vi "ERD Send Receive Example.vi"() -> ()   [LabVIEW 2016]
uses:
  Save File/File Setup (Public)/Type Definition/Save File DOE LabView Program.ctl
  type defs/ERD Read Data Out.ctl
  type defs/ERD Read Data In.ctl
  type defs/Data Type.ctl
  type defs/Source_Destination.ctl
  <vilib>/Utility/file.llb/Write To Spreadsheet File (string).vi
  library/GEA2_Toolkit.lvlib
  Save File/File Setup.lvlib
panel:
  out "Output Data Send":T1[](array[typedef]) {"ERD Number" format="%.0x"}
  in  "ERD to Send":T2[](array[typedef]) {"ERD Number" format="%.0x"}
  in  "Read ERD 2":bool
  in  "Add Date and Time":bool=TRUE
  out "Rate":dbl
  in  "#ERDs per message":i32=15
  out "ERD Data Out":T1[](array[typedef]) {"ERD Number" format="%.0x"}
  in  "ERD to Read":T2[](array[typedef]) {"ERD Number" format="%.0x"}
  out "Output Data Read":T1[](array[typedef]) {"ERD Number" format="%.0x"}
  in  "Read ERD":bool
  in  "Start Test":bool
  in  "Path":path
  in  "LV Program":T4=enum."HEWH"
  in  "Disable Classic GEA2":bool
  in  "Disable Electronic Mixing Valve (EMV) List":bool
  in  "Disable ERD":bool
  in  "Board Index":i32
  out "HEWH Appliance Data":string[][](array[string])
  in  "stop":bool
  # "HEWH Wifi Module\n0x600F - 01 Off\n0x600F - 00 On"
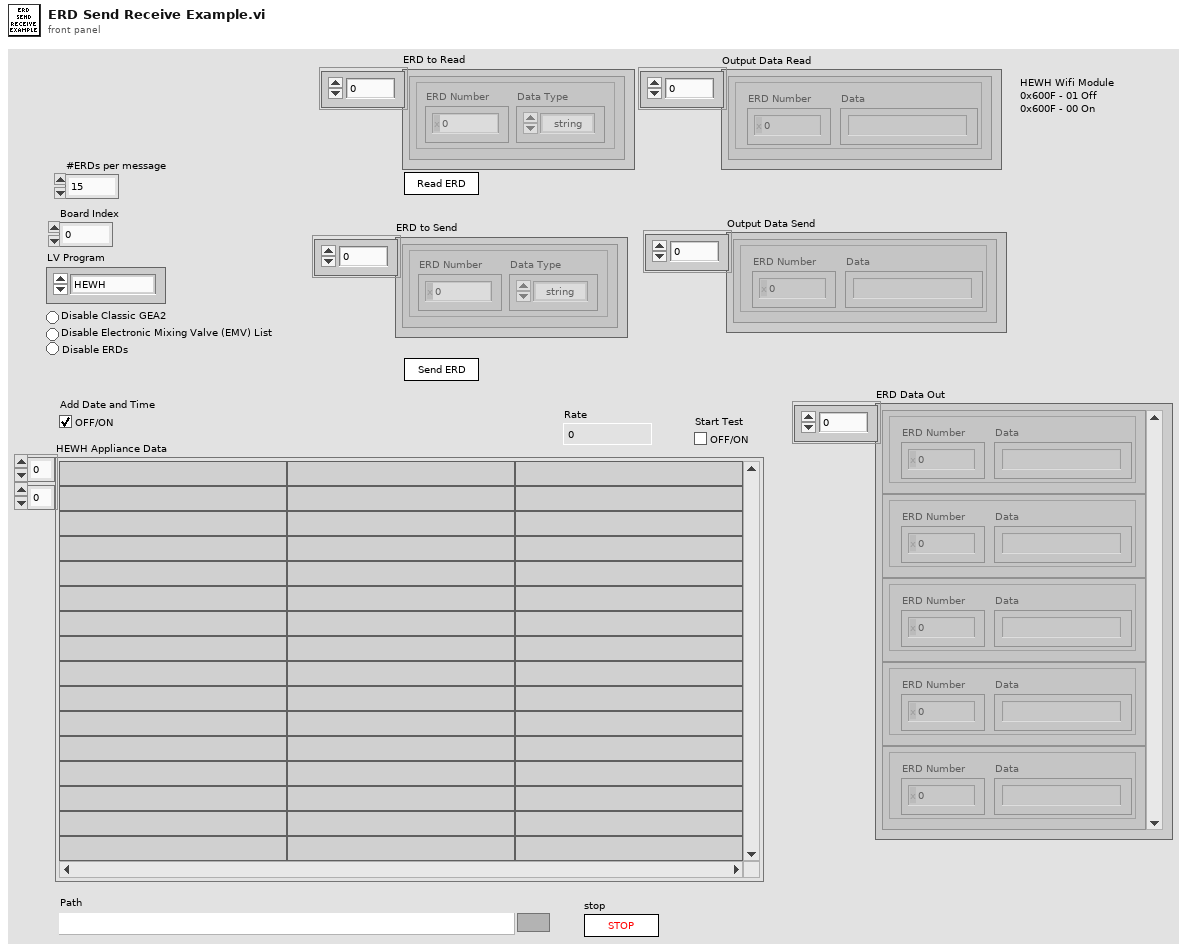
[diagram p1: front panel]
types:
  T1 = typedef "GEA2_Toolkit.lvlib/ERD Read Data Out.ctl" = cluster{"ERD Number":u16, "Data":string}
  T2 = typedef "GEA2_Toolkit.lvlib/ERD Read Data In.ctl" = cluster{"ERD Number":u16, "Data Type":T3}
  T3 = typedef "GEA2_Toolkit.lvlib/Data Type.ctl" = enum16{"string", "boolean", "uint8_t", "uint16_t", "uint32_t", "uint64_t"}
  T4 = typedef "File Setup.lvlib/Save File DOE LabView Program.ctl" = enum16{"No Name Found", "DOE Stand", "Dishwasher Kitchen", "Portable Stand", "HEWH", "Dryer", "Dryer WILT", "HCC", "PRAT", "HEWH RLT"}
  T5 = typedef "GEA2_Toolkit.lvlib/Source_Destination.ctl" = cluster{"Source":u8, "Destination":u8}
  T6 = enum32{"invalid app kind", "Development System", "Run Time System", "Student Edition", "Embedded LabVIEW", "Evaluation", "Custom"}
  T7 = enum32{"Invalid", "Standard", "Closed", "Hidden", "Minimized", "Maximized"}
  T8 = cluster{"Core":cluster{"Current VI Reference":refnum<vi>, "Close Panel on Exit?":bool}, "HEWH Appliance Data":string[][]}
  T9 = cluster{"Current VI Reference":refnum<vi>, "Close Panel on Exit?":bool}
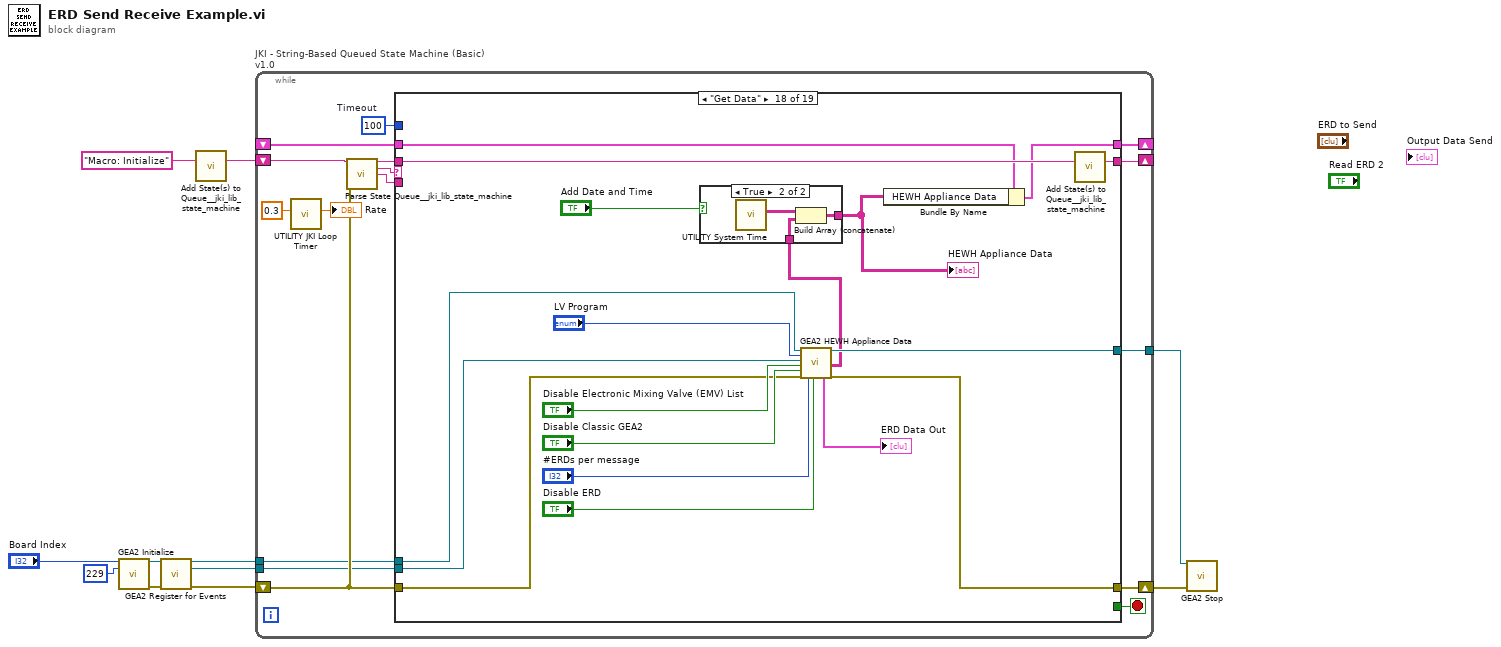
[diagram p0: block diagram]
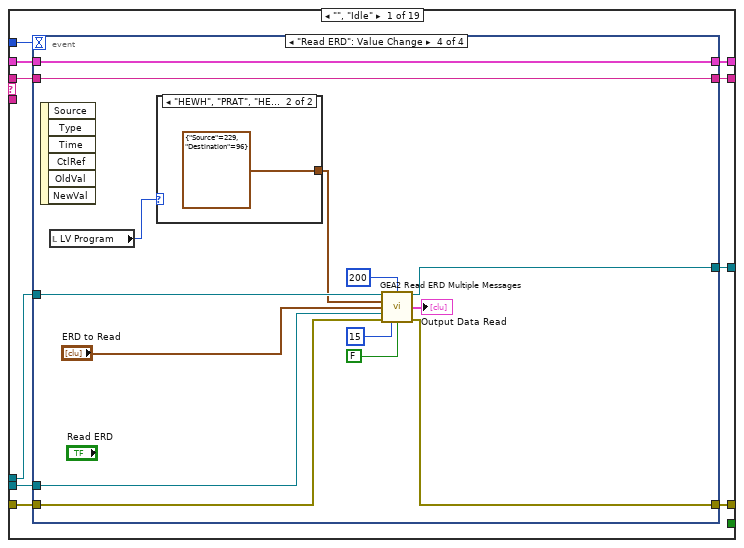
[diagram p2: hidden frame]
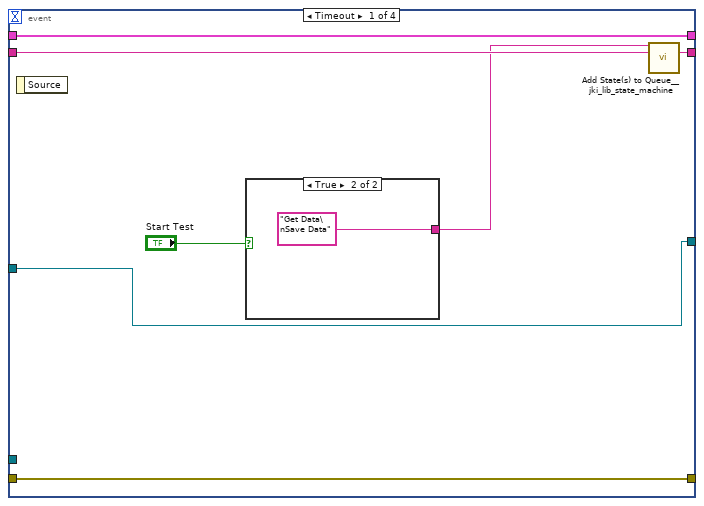
[diagram p3: hidden frame]
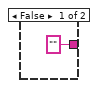
[diagram p4: hidden frame]
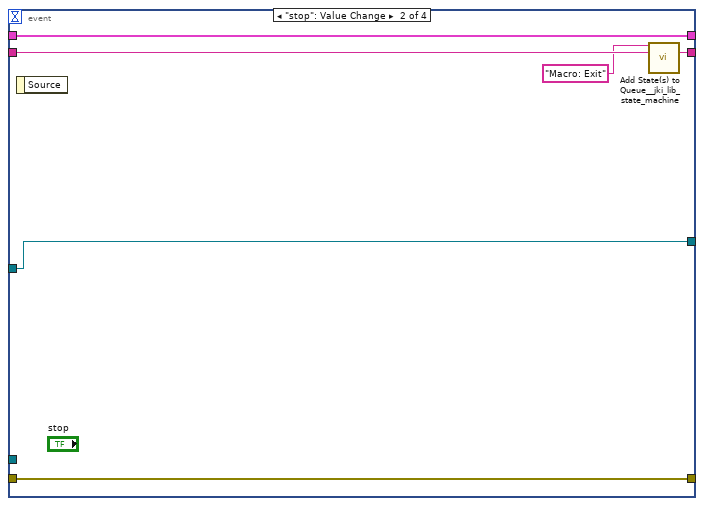
[diagram p5: hidden frame]
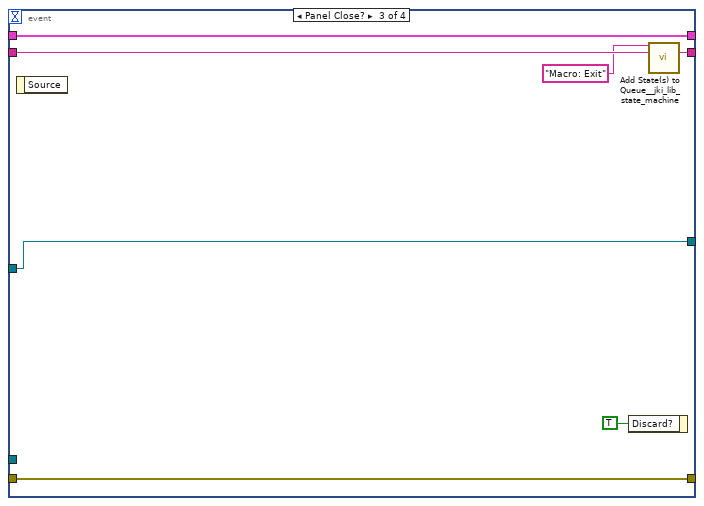
[diagram p6: hidden frame]
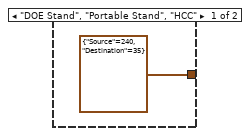
[diagram p7: hidden frame]
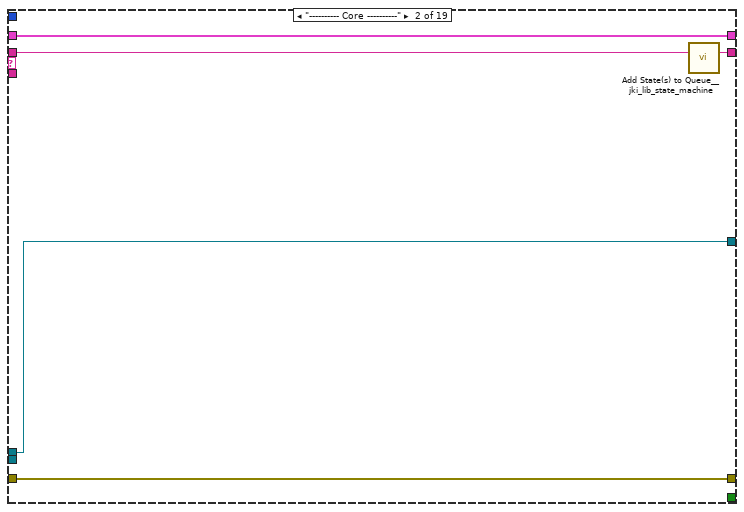
[diagram p8: hidden frame]
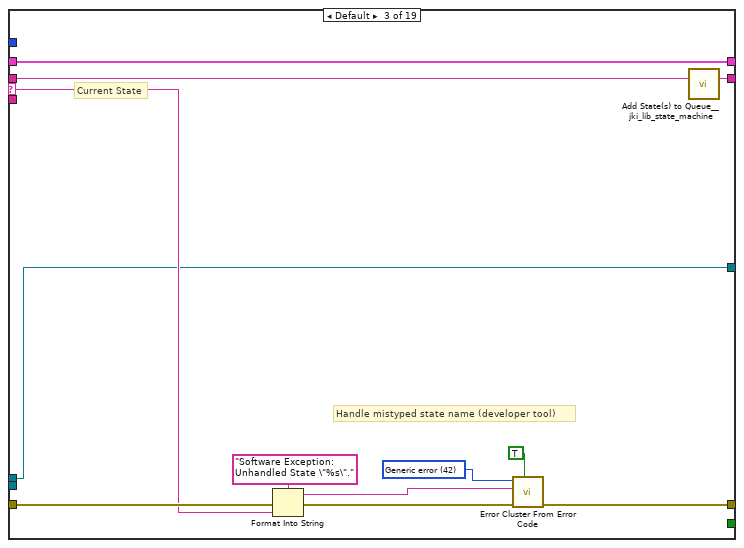
[diagram p9: hidden frame]
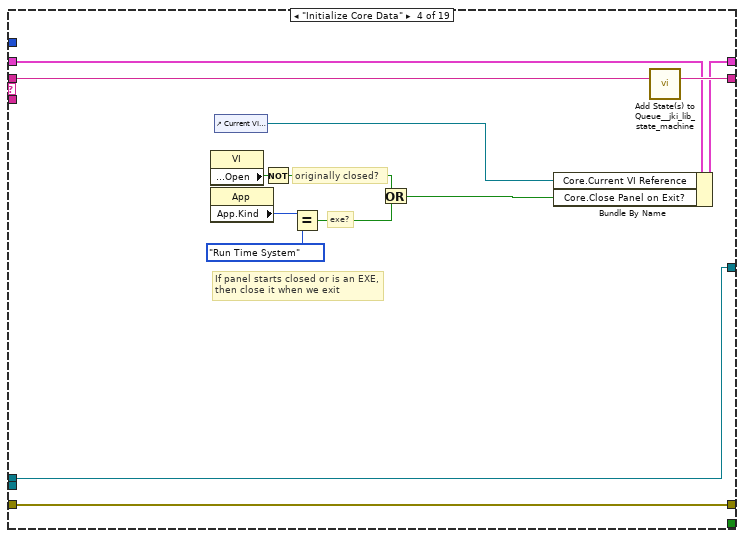
[diagram p10: hidden frame]
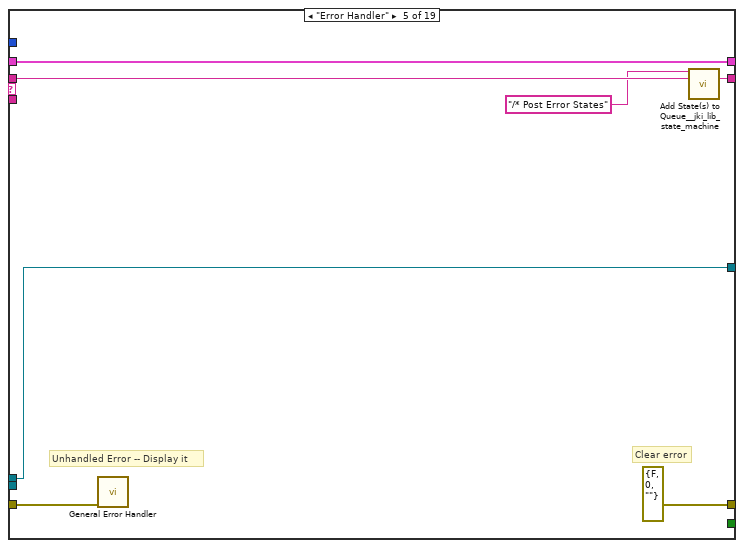
[diagram p11: hidden frame]
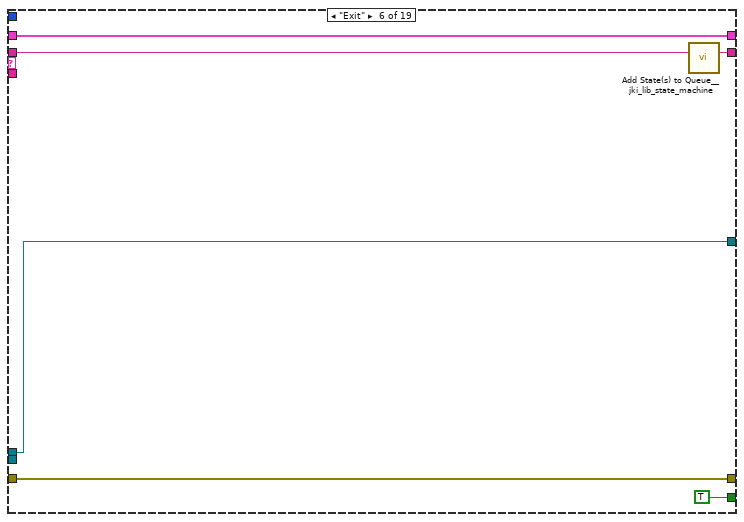
[diagram p12: hidden frame]
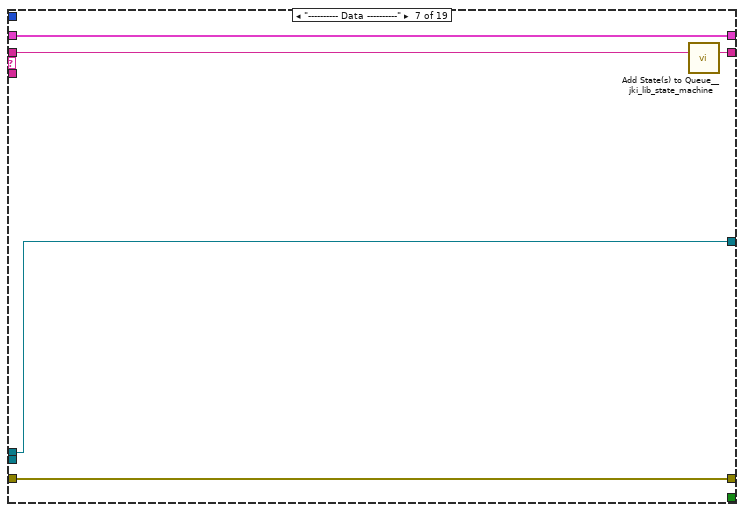
[diagram p13: hidden frame]
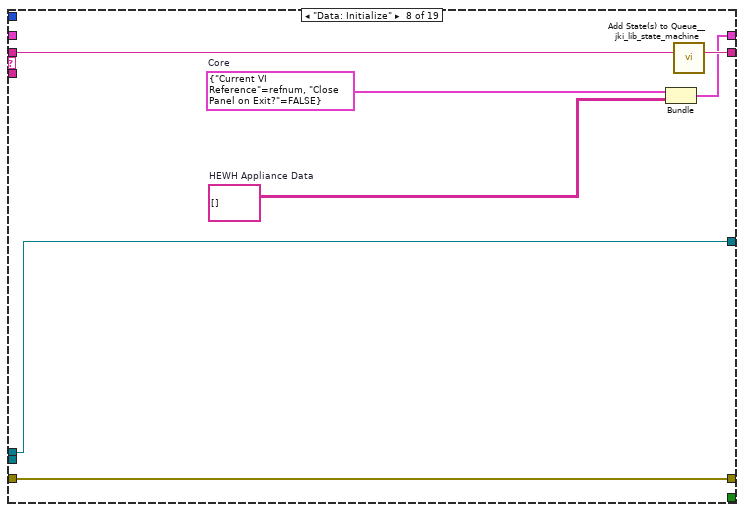
[diagram p14: hidden frame]
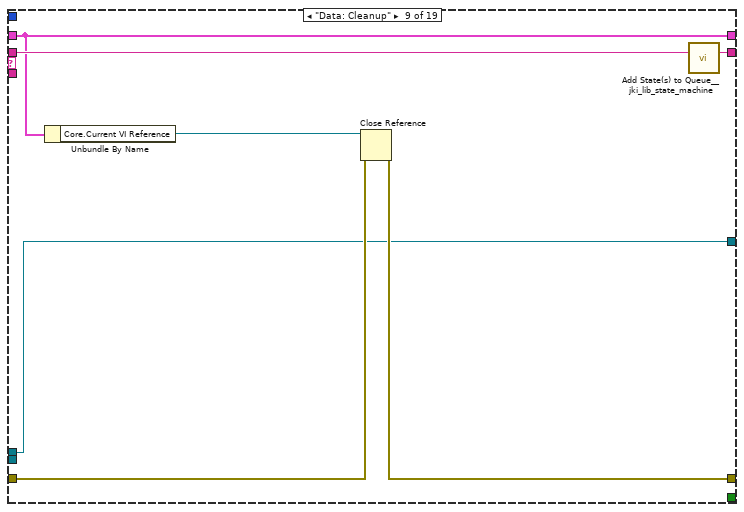
[diagram p15: hidden frame]
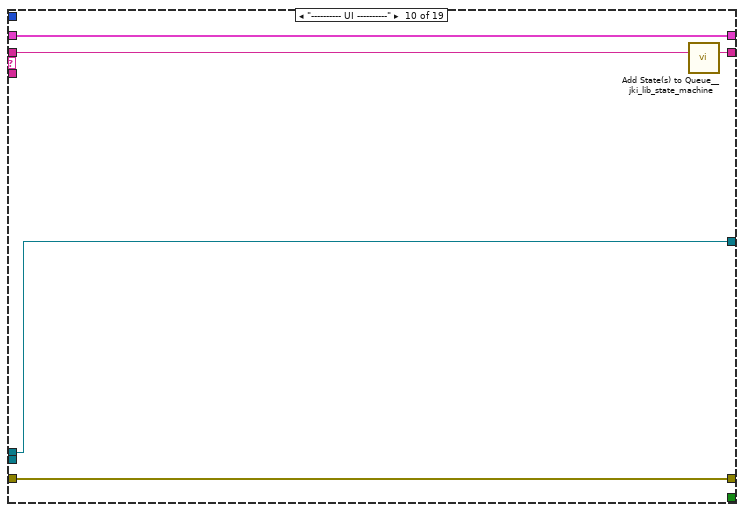
[diagram p16: hidden frame]
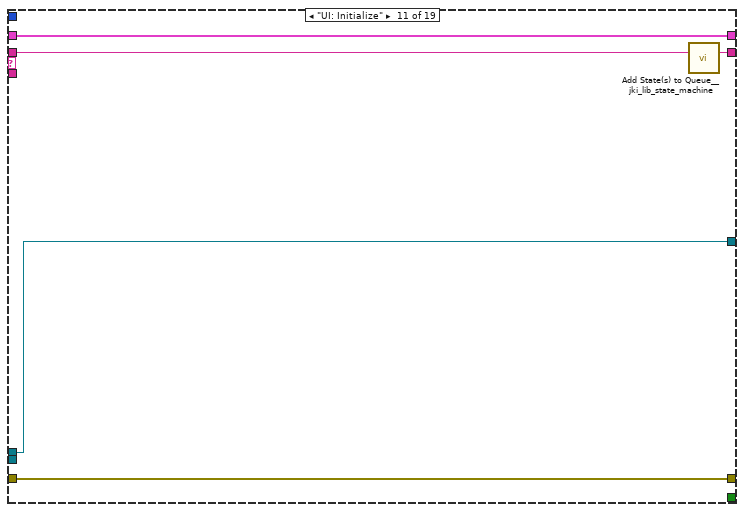
[diagram p17: hidden frame]
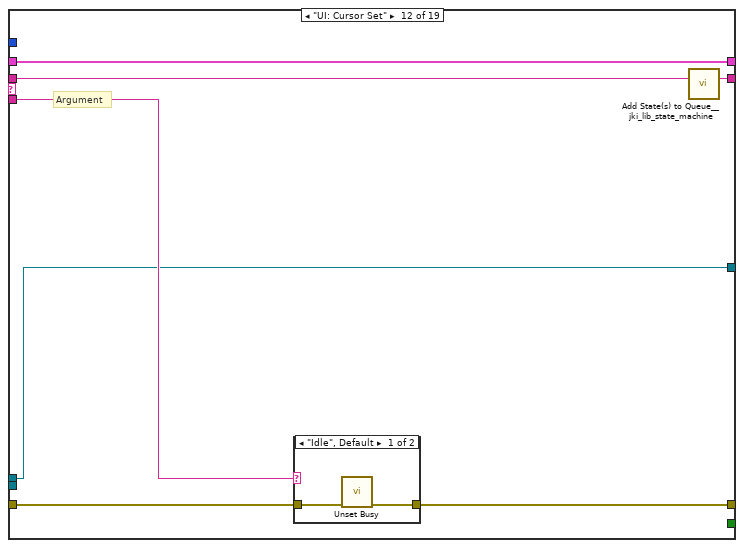
[diagram p18: hidden frame]
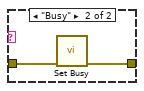
[diagram p19: hidden frame]
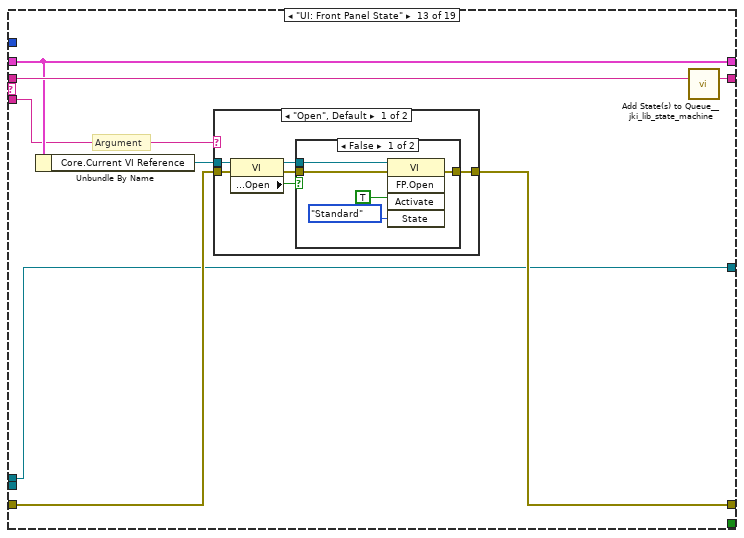
[diagram p20: hidden frame]
diagram:
  n1 = call "GEA2 Initialize.vi"("Board Index"="Board Index", "Source Address"=u8 229) -> ("GEA2 Reference Out"=w8:refnum<k24>, "error out"=w9:errorcluster)  [unwired: 11 in, 1 out]
  n2 = call "GEA2 Register for Events.vi"("GEA2 Reference In"=w8, "Error In"=w9) -> ("GEA2 Reference Out"=w3:refnum<k24>, "GEA2 Event Registration"=w2:refnum<event-registration>, "Error Out"=w5:errorcluster)  [unwired: 11 in]
  n3 = call <vilib>:"Add State(s) to Queue__jki_lib_state_machine.vi"("State(s) in (\"\")"="Macro: Initialize") -> ("States Out"=w7:string)  [unwired: 14 in]
  n4 = while "JKI - String-Based Queued State Machine (Basic) v1.0" {
    shift-right: [w20] -> _
    shift-left: _ -> [w19]
    shift-right: [w23] -> w4
    shift-left: w5 -> [w17]
    shift-right: [w22] -> _
    shift-left: w7 -> [w24]
    tunnel: w3 -> [w16]
    tunnel: w2 -> [w15]
    tunnel: [w14] -> w1
    stop <- w21 stop-if-true
    w18 = 100  # Timeout
    n5 = call "UTILITY JKI Loop Timer.vi"("K(0.3)"=0.3) -> ("Rate"=→"Rate":dbl)  [unwired: 9 in, 1 out]
    n6 = call <vilib>:"Parse State Queue__jki_lib_state_machine.vi"("State Queue"=w24, "Error In (no error)"=w17) -> ("Remaining States"=w26:string, "Current State"=w27:string, "Arguments"=w25:string)  [unwired: 11 in]
    n7 = case shown="\"Get Data\"" w27 {
      selector: w27 -> [_ _ w82 _ _ _ _ _ _ _ _ _ _ _ _ _ _ _ _]
      tunnel: w26 -> [w37 w80 w86 w105 w112 w118 w123 w130 w137 w142 w147 w154 w166 w193 w199 w210 w215 w233 w246]
      tunnel: w25 -> [_ _ _ _ _ _ _ _ _ _ _ w149 w160 _ _ _ _ _ _]
      tunnel: w19 -> [w35 w77 w84 w96 w109 w116 w120 _ w132 w139 w145 w152 w162 w190 w196 w207 w212 w225 w241]
      tunnel: [w34 w78 w88 w102 errorcluster {"status"=FALSE, "code"=0, "source"=""} ("error out") w115 w121 w127 w133 w140 w144 w150 w163 w191 w197 w208 w213 w226 w242] -> w23
      tunnel: w17 -> [w33 w78 w87 w102 w108 w115 w121 w127 w134 w140 w144 w151 w164 w191 w197 w208 w213 w227 w243]
      tunnel: [w36 w79 w85 w104 w111 w117 w122 w129 w136 w141 w146 w153 w165 w192 w198 w209 w214 w232 w245] -> w22
      tunnel: [_ _ _ _ _ TRUE _ _ _ _ _ _ _ _ _ _ _ _ _] -> w21
      tunnel: [w32 w77 w84 w103 w109 w116 w120 w128 w132 w139 w145 w152 w162 w190 w196 w207 w212 w224 w241] -> w20
      tunnel: w18 -> [w31 _ _ _ _ _ _ _ _ _ _ _ _ _ _ _ _ _ _]
      tunnel: w16 -> [w30 w76 w81 w93 w106 w113 w119 w124 w131 w138 w143 w148 w159 w189 w194 w200 w211 w223 w239]
      tunnel: w15 -> [w29 _ _ _ _ _ _ _ _ _ _ _ _ _ _ _ _ w222 _]
      tunnel: [w28 w76 w81 w93 w106 w113 w119 w124 w131 w138 w143 w148 w159 w189 w194 w200 w211 w221 w239] -> w14
      frame "", "Idle" {
        n8 = event shown="[3] \"Read ERD\": Value Change" {
          selector: _ -> [_ _ _ _]
          dyn-events: _ -> [_ _ _ _]
          timeout: w31 -> [_ _ _ _]
          tunnel: w37 -> [w44 w52 w59 w72]
          tunnel: [w43 w51 w58 w72] -> w36
          tunnel: w35 -> [w41 w49 w56 w73]
          tunnel: [w42 w50 w57 w61] -> w34
          tunnel: w33 -> [w42 w50 w57 w62]
          tunnel: [w41 w49 w56 w73] -> w32
          tunnel: w30 -> [w38 w47 w53 w66]
          tunnel: w29 -> [_ _ _ w65]
          tunnel: [w38 w47 w53 w63] -> w28
          event Timeout {
            n9 = event-data() -> ()  [unwired: 1 in, 1 out]
            n10 = case shown="True" "Start Test" {
              tunnel: ["" ("State(s) in Front (\"\")") "Get Data\nSave Data" ("State(s) in Front (\"\")")] -> w40
              frame False {
              }
              frame True {
              }
            }
            n11 = call <vilib>:"Add State(s) to Queue__jki_lib_state_machine.vi"("State(s) in Front (\"\")"=w40, "State(s) in (\"\")"=w44) -> ("States Out"=w43:string)  [unwired: 13 in]
          }
          event "stop": Value Change {
            n12 = event-data() -> ()  [unwired: 1 in, 1 out]
            n13 = call <vilib>:"Add State(s) to Queue__jki_lib_state_machine.vi"("State(s) in Front (\"\")"="Macro: Exit", "State(s) in (\"\")"=w52) -> ("States Out"=w51:string)  [unwired: 13 in]
          }
          event Panel Close? {
            n14 = event-data() -> ()  [unwired: 1 in, 1 out]
            n15 = event-data("Discard?"=TRUE) -> ()  [unwired: 1 in, 1 out]
            n16 = call <vilib>:"Add State(s) to Queue__jki_lib_state_machine.vi"("State(s) in Front (\"\")"="Macro: Exit", "State(s) in (\"\")"=w59) -> ("States Out"=w58:string)  [unwired: 13 in]
          }
          event "Read ERD": Value Change {
            n17 = event-data() -> ()  [unwired: 1 in, 6 out]
            n18 = local read "LV Program"() -> (w60:T4)
            n19 = case shown="\"HEWH\", \"PRAT\", \"HEWH RLT\", Default" w60 {
              tunnel: [T5 {"Source"=240, "Destination"=35} ("GEA Inputs") T5 {"Source"=229, "Destination"=96} ("GEA Inputs")] -> w64
              frame "DOE Stand", "Portable Stand", "HCC" {
              }
              frame "HEWH", "PRAT", "HEWH RLT", Default {
              }
            }
            n20 = call "GEA2 Read ERD Multiple Messages.vi"("GEA2 Reference In"=w66, "Read Timeout (ms)"=u32 200, "GEA Inputs"=w64, "Read ERD List"="ERD to Read", "GEA2 Event Registration"=w65, "Error In"=w62, "#ERDs per message"=15, "Verify ERD Response?"=FALSE) -> ("GEA2 Reference Out"=w63:refnum<k24>, "ERD Data Out"=→"Output Data Read":T1[], "Error Out"=w61:errorcluster)  [unwired: 3 in, 2 out]
          }
        }
      }
      frame "---------- Core ----------" {
        n21 = call <vilib>:"Add State(s) to Queue__jki_lib_state_machine.vi"("State(s) in (\"\")"=w80) -> ("States Out"=w79:string)  [unwired: 14 in]
      }
      frame Default {
        w91 = 42 items=["No error", "Argument error", "Memory is full", "Out of zone", "End of file", "File already open", "Generic file I/O error", "File not found", "File permission error", "Disk is full", "Duplicate path", "Too many files open", "System feature not enabled", "Resource file not found", "Cannot add resource", "Resource not found", "Image not found", "Image memory error", "Pen does not exist", "Config type invalid", "Config token not found", "Config parse error", "Config memory error", "Bad external code format", "Bad external code offset", "External code not present", "Null window", "Destroy window error", "Null menu", "Print aborted", "Bad print record", "Print driver error", "Windows error during printing", "Memory error during printing", "Print dialog error", "Generic print error", "Invalid device refnum", "Device not found", "Device parameter error", "Device unit error", "Cannot open device", "Device call aborted", "Generic error", "Cancelled by user", "Object ID too low", "Object ID too high", "Object not in heap", "Unknown heap", "Unknown object (invalid DefProc)", "Unknown object (DefProc not in table)", "Message out of range", "Invalid (null) method", "Unknown message", "Manager call not supported", "Bad address", "Network operation in progress", "Network operation timed out", "Connection is busy", "Network attribute not supported", "Network error", "Address in use", "System out of memory", "Connection aborted", "Connection refused", "Not connected", "Already connected", "Connection closed", "Initialization error (interapplication manager)", "Bad occurrence", "Wait on unbound occurrence handler", "Occurrence queue overflow", "Datalog type conflict", "Unused", "Unrecognized type (interapplication manager)", "Memory corrupt", "Failed to make temporary DLL", "Old CIN version", "Drag socket not found", "Failed to load drop-object", "Failed to register OLE object", "Failed to release OLE object", "Format specifier type mismatch", "Unknown format specifier", "Too few format specifiers", "Too many format specifiers", "Scan failed", "Newer CIN version", "Error converting to variant", "Runtime menu error", "Password tampered", "Variant attribute not found", "Incompatible variant data type", "Event data is not available", "Event Store is not present", "Occurrence is not found", "Event Queue is not created", "Event info is not available", "Refnum passed is NULL", "Error retrieving Class GUID", "Error retrieving CoClass GUID", "Error retrieving TypeLib GUID.", "Bad built application magic bytes.", "Specific driver is different from the specific driver associated with the Logical Name.", "There is no session opened to the class driver.", "Max Error", "MAX - Error with config objects", "MAX - Error loading configuration", "MAX - Group not supported"]
        # "Current State"
        # "Handle mistyped state name (developer tool)"
        n22 = Format Into String(format string="Software Exception: Unhandled State \"%s\"." ("message"), error in=w87, w82) -> (resulting string=w90:string, error out=w89:errorcluster)  [unwired: 1 in]
        n23 = call <vilib>:"Error Cluster From Error Code.vi"("show call chain? (False)"=TRUE, "error in (no error)"=w89, "error message (\"\")"=w90, "error code (0)"=w91) -> ("error out"=w88:errorcluster)  [unwired: 5 in]
        n24 = call <vilib>:"Add State(s) to Queue__jki_lib_state_machine.vi"("State(s) in (\"\")"=w86) -> ("States Out"=w85:string)  [unwired: 14 in]
      }
      frame "Initialize Core Data" {
        # "originally closed?"
        # "exe?"
        # "If panel starts closed or is an EXE, then close it when we exit"
        n25 = property class="VI"() -> ("Front Panel.Open"=w101:bool)  [unwired: 2 in, 2 out]
        n26 = property class="App"() -> ("App.Kind"=w100:T6)  [unwired: 2 in, 2 out]
        n27 = control-ref of="Current VI Reference"() -> (w94:refnum<vi>)
        n28 = Not(x=w101) -> (.not. x?=w98:bool)
        n29 = Equal?(x=w100, y=T6."Run Time System" ("Application:Kind")) -> (x = y?=w97:bool)
        n30 = Or(x=w98, y=w97) -> (x .or. y?=w95:bool)
        n31 = Bundle By Name(cluster=w96, "Core.Current VI Reference"=w94, "Core.Close Panel on Exit?"=w95) -> (w103:T8)
        n32 = call <vilib>:"Add State(s) to Queue__jki_lib_state_machine.vi"("State(s) in (\"\")"=w105) -> ("States Out"=w104:string)  [unwired: 14 in]
      }
      frame "Error Handler" {
        # "Unhandled Error -- Display it"
        # "Clear error"
        n33 = call <vilib>:"General Error Handler.vi"("error in (no error)"=w108) -> ()  [unwired: 10 in, 5 out]
        n34 = call <vilib>:"Add State(s) to Queue__jki_lib_state_machine.vi"("State(s) in Front (\"\")"="/* Post Error States", "State(s) in (\"\")"=w112) -> ("States Out"=w111:string)  [unwired: 13 in]
      }
      frame "Exit" {
        n35 = call <vilib>:"Add State(s) to Queue__jki_lib_state_machine.vi"("State(s) in (\"\")"=w118) -> ("States Out"=w117:string)  [unwired: 14 in]
      }
      frame "---------- Data ----------" {
        n36 = call <vilib>:"Add State(s) to Queue__jki_lib_state_machine.vi"("State(s) in (\"\")"=w123) -> ("States Out"=w122:string)  [unwired: 14 in]
      }
      frame "Data: Initialize" {
        w125 = string[][] []  # HEWH Appliance Data
        w126 = T9 {"Current VI Reference"=refnum, "Close Panel on Exit?"=FALSE}  # Core
        n37 = Bundle("Core"=w126, "HEWH Appliance Data"=w125) -> (w128:T8)  [unwired: 1 in]
        n38 = call <vilib>:"Add State(s) to Queue__jki_lib_state_machine.vi"("State(s) in (\"\")"=w130) -> ("States Out"=w129:string)  [unwired: 14 in]
      }
      frame "Data: Cleanup" {
        n39 = Unbundle By Name(w132) -> ("Core.Current VI Reference"=w135:refnum<vi>)
        n40 = Close Reference(reference=w135, error in (no error)=w134) -> (error out=w133:errorcluster)
        n41 = call <vilib>:"Add State(s) to Queue__jki_lib_state_machine.vi"("State(s) in (\"\")"=w137) -> ("States Out"=w136:string)  [unwired: 14 in]
      }
      frame "---------- UI ----------" {
        n42 = call <vilib>:"Add State(s) to Queue__jki_lib_state_machine.vi"("State(s) in (\"\")"=w142) -> ("States Out"=w141:string)  [unwired: 14 in]
      }
      frame "UI: Initialize" {
        n43 = call <vilib>:"Add State(s) to Queue__jki_lib_state_machine.vi"("State(s) in (\"\")"=w147) -> ("States Out"=w146:string)  [unwired: 14 in]
      }
      frame "UI: Cursor Set" {
        # "Argument"
        n44 = case shown="\"Idle\", Default" w149 {
          tunnel: w151 -> [w156 w158]
          tunnel: [w155 w157] -> w150
          frame "Idle", Default {
            n45 = call <vilib>:"Unset Busy.vi"("error in (no error)"=w156) -> ("error out"=w155:errorcluster)  [unwired: 10 in]
          }
          frame "Busy" {
            n46 = call <vilib>:"Set Busy.vi"("error in (no error)"=w158) -> ("error out"=w157:errorcluster)  [unwired: 9 in, 1 out]
          }
        }
        n47 = call <vilib>:"Add State(s) to Queue__jki_lib_state_machine.vi"("State(s) in (\"\")"=w154) -> ("States Out"=w153:string)  [unwired: 14 in]
      }
      frame "UI: Front Panel State" {
        # "Argument"
        n48 = Unbundle By Name(w162) -> ("Core.Current VI Reference"=w161:refnum<vi>)
        n49 = case shown="\"Open\", Default" w160 {
          tunnel: w164 -> [w170 w183]
          tunnel: [w172 w184] -> w163
          tunnel: w161 -> [w171 w181]
          frame "Open", Default {
            n50 = property class="VI"(reference=w171, error in=w170) -> (reference out=w168:refnum<vi>, error out=w169:errorcluster, "Front Panel.Open"=w167:bool)
            n51 = case shown="False" w167 {
              tunnel: [w175 w178] -> w172
              tunnel: w169 -> [w174 w178]
              tunnel: w168 -> [w173 _]
              frame False {
                n52 = invoke class="VI" method="FP.Open"(reference=w173, error in=w174, "Activate"=TRUE, "State"=T7."Standard") -> (error out=w175:errorcluster)  [unwired: 1 in, 4 out]
              }
              frame True {
              }
            }
          }
          frame "Close" {
            n53 = property class="VI"(reference=w181, error in=w183) -> (reference out=w180:refnum<vi>, error out=w182:errorcluster, "Front Panel.Open"=w179:bool)
            n54 = case shown="True" w179 {
              tunnel: [w185 w188] -> w184
              tunnel: w182 -> [w185 w187]
              tunnel: w180 -> [_ w186]
              frame False {
              }
              frame True {
                n55 = invoke class="VI" method="FP.Close"(reference=w186, error in=w187) -> (error out=w188:errorcluster)  [unwired: 1 in, 2 out]
              }
            }
          }
        }
        n56 = call <vilib>:"Add State(s) to Queue__jki_lib_state_machine.vi"("State(s) in (\"\")"=w166) -> ("States Out"=w165:string)  [unwired: 14 in]
      }
      frame "---------- Macro ----------" {
        n57 = call <vilib>:"Add State(s) to Queue__jki_lib_state_machine.vi"("State(s) in (\"\")"=w193) -> ("States Out"=w192:string)  [unwired: 14 in]
      }
      frame "Macro: Initialize" {
        w195 = "Data: Initialize\nInitialize Core Data\nUI: Initialize\nUI: Front Panel State >> Open"  # Data: Initialize Initialize Core Data UI: Initialize UI: Front Panel State >> Open
        n58 = call <vilib>:"Add State(s) to Queue__jki_lib_state_machine.vi"("State(s) in Front (\"\")"=w195, "State(s) in (\"\")"=w199) -> ("States Out"=w198:string)  [unwired: 13 in]
      }
      frame "Macro: Exit" {
        n59 = Unbundle By Name(w207) -> ("Core.Close Panel on Exit?"=w206:bool)
        n60 = Select(t="UI: Front Panel State >> Close", s=w206, f="") -> (s? t:f=w203:string)
        n61 = call <vilib>:"Add State(s) to Queue__jki_lib_state_machine.vi"("State(s) in (\"\")"=w203, "State(s) at Back (\"\")"="Data: Cleanup\nExit") -> ("States Out"=w201:string)  [unwired: 13 in]
        n62 = call <vilib>:"Add State(s) to Queue__jki_lib_state_machine.vi"("State(s) in Front (\"\")"=w201, "State(s) in (\"\")"=w210) -> ("States Out"=w209:string)  [unwired: 13 in]
      }
      frame "---------- New Category ----------" {
        n63 = call <vilib>:"Add State(s) to Queue__jki_lib_state_machine.vi"("State(s) in (\"\")"=w215) -> ("States Out"=w214:string)  [unwired: 14 in]
      }
      frame "Get Data" {
        n64 = call "GEA2 HEWH Appliance Data.vi"(".NET Refnum in"=w223, "LV Program"="LV Program", "GEA2 Event Registration In"=w222, "Disable Electronic Mixing Valve (EMV) List"="Disable Electronic Mixing Valve (EMV) List", "Disable Classic GEA2"="Disable Classic GEA2", "error in (no error)"=w227, "#ERDs per message"="#ERDs per message", "Disable ERD A"="Disable ERD") -> ("ERD Data Out"=→"ERD Data Out":T1[], ".NET Refnum out"=w221:refnum<k24>, "HEWH Appliance Data ERD"=w218:string[][], "error out"=w226:errorcluster)  [unwired: 5 in, 3 out]
        n65 = case shown="True" "Add Date and Time" {
          tunnel: w218 -> [w234 w236]
          tunnel: [w234 w235] -> w217
          frame False {
          }
          frame True {
            n66 = call "UTILITY System Time.vi"() -> ("Date & Time"=w237:string[][])  [unwired: 10 in, 1 out]
            n67 = Build Array (concatenate)(w237, w236) -> (w235:string[][])
          }
        }
        "HEWH Appliance Data" <- w217
        n68 = Bundle By Name(cluster=w225, "HEWH Appliance Data"=w217) -> (w224:T8)
        n69 = call <vilib>:"Add State(s) to Queue__jki_lib_state_machine.vi"("State(s) in (\"\")"=w233) -> ("States Out"=w232:string)  [unwired: 14 in]
      }
      frame "Save Data" {
        n70 = Unbundle By Name(w241) -> ("HEWH Appliance Data"=w240:string[][])
        n71 = First Call?() -> (First Call?: T/F=w244:bool)
        n72 = case shown="False" w244 {
          tunnel: "Path" -> [w250 w258]
          tunnel: w240 -> [w253 w256]
          tunnel: w243 -> [w247 w254]
          tunnel: [w247 w254] -> w242
          frame False {
            n73 = Index Array(array=w253, index (col)=1 ("disabled index (col)")) -> (element=w251:string[])  [unwired: 1 in]
            n74 = call-poly <vilib>:"Write To Spreadsheet File.vi"("delimiter (\\t)"="," ("delimiter (\\t)"), "append to file? (new file:F)"=TRUE, "1D data"=w251, "file path (dialog if empty)"=w250) -> ()  [unwired: 4 in, 1 out]
          }
          frame True {
            n75 = Transpose 2D Array(2D array=w256) -> (transposed array=w255:string[][])
            n76 = call-poly <vilib>:"Write To Spreadsheet File.vi"("delimiter (\\t)"="," ("delimiter (\\t)"), "2D data"=w255, "file path (dialog if empty)"=w258) -> ()  [unwired: 5 in, 1 out]
          }
        }
        n77 = call <vilib>:"Add State(s) to Queue__jki_lib_state_machine.vi"("State(s) in (\"\")"=w246) -> ("States Out"=w245:string)  [unwired: 14 in]
      }
    }
  }
  n78 = call "GEA2 Stop.vi"("GEA2 Reference Out"=w1, "Error In"=w4) -> ()  [unwired: 13 in, 1 out]
